vi "Process-Stop Logic.vi"(11 "Wait on post-processing":refnum<k4>) -> (3 "Abort logging":bool)   [LabVIEW 2013]
uses:
  Typedefs/Read Write Enum.ctl
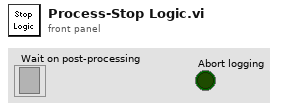
[diagram p1: front panel]
types:
  T1 = typedef "Read Write Enum.ctl" = enum16{"Read", "Write"}
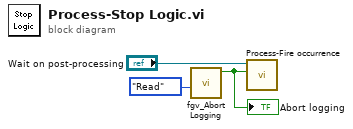
[diagram p0: block diagram]
diagram:
  n1 = call "fgv_Abort Logging.vi"("Function"=Read_Write_Enum."Read") -> ("Abort logging"=w2:bool)  [unwired: 9 in, 1 out]
  "Abort logging" <- w2
  n2 = call "Process-Fire occurrence.vi"("Abort logging"=w2, "Wait on post-processing"="Wait on post-processing") -> ()  [unwired: 10 in]
